vi "closeCAM.vi"(8 "error in (no error)":errorcluster, 11 "Input cluster":T1) -> (0 "error out":errorcluster, 3 "Output cluster":T1)   [LabVIEW 2020]
doc: "Close opened camera session."
uses:
  controls/StateMachineVariables.ctl
  <vilib>/vision/Avi.llb/IMAQ AVI2 Refnum.ctl
  <vilib>/userDefined/High Color/IMAQdx.ctl
  <vilib>/vision/Deep Learning.llb/IMAQ DL Model Refnum.ctl
  <vilib>/vision/Image Controls.llb/IMAQ Image.ctl
  <vilib>/vision/driver/NI_Vision_Acquisition_Software.lvlib
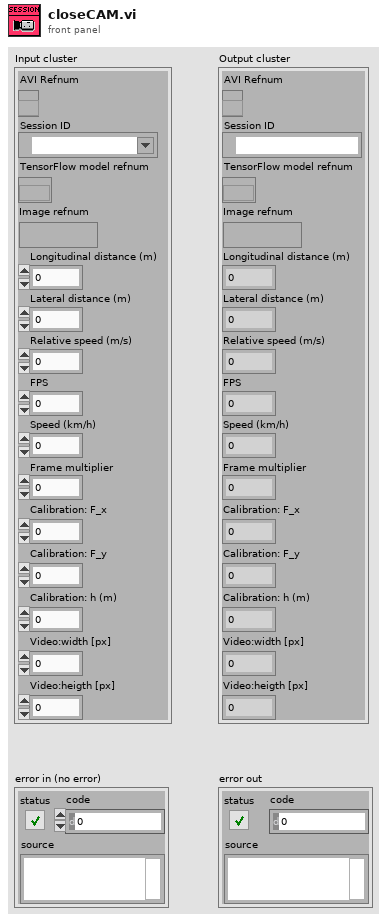
[diagram p1: front panel]
types:
  T1 = typedef "StateMachineVariables.ctl" = cluster{"AVI Refnum":T2, "Session ID":T3, "TensorFlow model refnum":T4, "Image refnum":T5, "Longitudinal distance (m)":dbl, "Lateral distance (m)":dbl, "Relative speed (m/s)":dbl, "FPS":dbl, "Speed (km/h)":dbl, "Frame multiplier":u32, "Calibration: F_x":dbl, "Calibration: F_y":dbl, "Calibration: h (m)":dbl, "Video:width [px]":i32, "Video:heigth [px]":i32}
  T2 = typedef "IMAQ AVI2 Refnum.ctl" = refnum<k20>
  T3 = typedef "IMAQdx.ctl" = refnum<k21>
  T4 = typedef "IMAQ DL Model Refnum.ctl" = refnum<k20>
  T5 = typedef "IMAQ Image.ctl" = refnum<image>
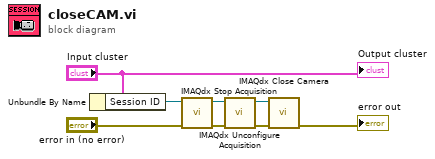
[diagram p0: block diagram]
diagram:
  n1 = Unbundle By Name("Input cluster") -> ("Session ID"=w8:T3)
  n2 = call <vilib>:"IMAQdx Stop Acquisition.vi"("error in"="error in (no error)", "Session In"=w8) -> ("error out"=w2:errorcluster, "Session Out"=w4:T3)  [unwired: 8 out]
  n3 = call <vilib>:"IMAQdx Unconfigure Acquisition.vi"("error in"=w2, "Session In"=w4) -> ("error out"=w1:errorcluster, "Session Out"=w3:T3)  [unwired: 8 out]
  n4 = call <vilib>:"IMAQdx Close Camera.vi"("error in"=w1, "Session In"=w3) -> ("error out"=→"error out":errorcluster)  [unwired: 9 out]
  "Output cluster" <- "Input cluster"
